vi "Read Exception Status.vi"(8 "error in":errorcluster, 11 "Modbus slave in":refnum<class "Modbus Slave.lvclass">) -> (0 "error out":errorcluster, 2 "exception status":u8, 3 "Modbus slave out":refnum<class "Modbus Slave.lvclass">)   [LabVIEW 2014, in "MyLib.lvlib" / "Modbus Slave.lvclass"]
doc: "Interface to reads any exception status set in the device. The exeption status is a set of 8 status bits, packed as a U8 integer. With third-party devices, this function should only be used if the device is a serial device, as the Modbus specification defines this as a serial-only function. However, this library includes support for this function regardless of the transport mechanism."
uses:
  Modbus Slave.lvclass
  Modbus Slave.lvclass/Modbus Slave.ctl
  Data Model/Device Data Model.lvclass
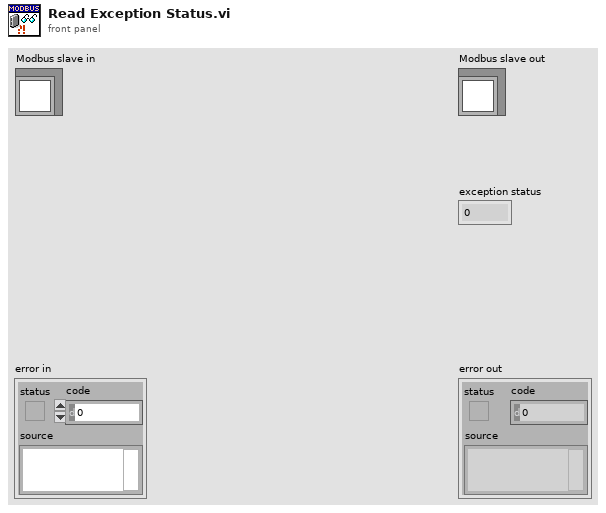
[diagram p1: front panel]
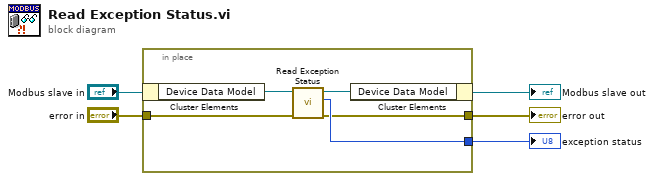
[diagram p0: block diagram]
diagram:
  n1 = in-place {
    in-place-border: [w10] -> w2
    in-place-border: [w9] -> w3
    in-place-border: "error in" -> [w8]
    n2 = in-place-cluster #1("Modbus slave in") -> ("Device Data Model"=w7:refnum<class "Device Data Model.lvclass">)
    n3 = call-dynamic "Read Exception Status.vi"("error in"=w8, "device data model in"=w7) -> ("error out"=w9:errorcluster, "exception status"=w10:u8, "device data model out"=w6:refnum<class "Device Data Model.lvclass">)  [unwired: 7 in]
    n4 = in-place-cluster #1("Device Data Model"=w6) -> (→"Modbus slave out":refnum<class "Modbus Slave.lvclass">)
  }
  "error out" <- w3
  "exception status" <- w2
